vi "TrimHourMin.vi"(11 "Time":timestamp format="%<%I:%M %p>T") -> (0 "hr+min":i32, 1 "minute(00-59)":i32, 3 "hour(00-23)":i32)   [LabVIEW 2011]
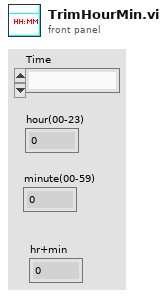
[diagram p1: front panel]
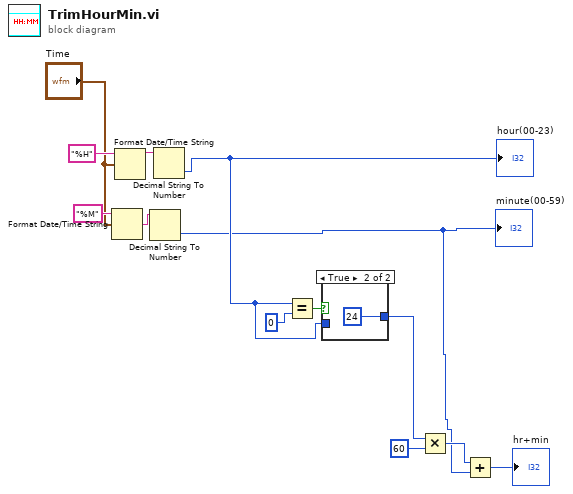
[diagram p0: block diagram]
diagram:
  n1 = Format Date/Time String(time format string (%c)="%M", seconds (now)="Time") -> (date/time string=w9:string)  [unwired: 1 in]
  n2 = Format Date/Time String(time format string (%c)="%H", seconds (now)="Time") -> (date/time string=w10:string)  [unwired: 1 in]
  n3 = Decimal String To Number(string=w9) -> (number=w1:i32)  [unwired: 2 in, 1 out]
  "minute(00-59)" <- w1
  n4 = Decimal String To Number(string=w10) -> (number=w3:i32)  [unwired: 2 in, 1 out]
  "hour(00-23)" <- w3
  n5 = Equal?(x=w3, y=0) -> (x = y?=w5:bool)
  n6 = case shown="True" w5 {
    tunnel: [w14 24] -> w2
    tunnel: w3 -> [w14 _]
    frame False {
    }
    frame True {
    }
  }
  n7 = Multiply(x=w2, y=60) -> (x*y=w7:i32)
  n8 = Add(x=w7, y=w1) -> (x+y=→"hr+min":i32)
